vi "Path - ResolveHostRoot.vi"(8 "error in (no error)":errorcluster) -> (0 "error out":errorcluster)   [LabVIEW 2026, in "Tests.lvlib"]
doc: "Update with test documentation"
uses:
  Tests.lvlib
  <vilib>/addons/_JKI Toolkits/Caraya/classes/Assert/Assert Equal Value_Variant.vi
  <vilib>/addons/_JKI Toolkits/Caraya/classes/Assert/Assert Error.vi
  <vilib>/addons/_JKI Toolkits/Caraya/classes/Test/Test.lvclass
  src/Lumberjack.lvlib
  <vilib>/addons/_JKI Toolkits/Caraya/classes/Assert/Assert.lvclass
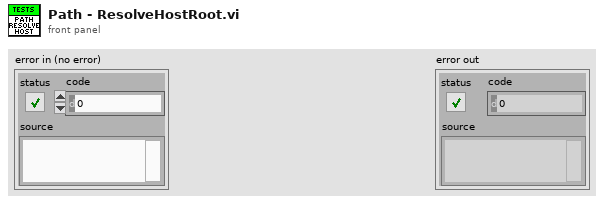
[diagram p1: front panel]
types:
  T1 = enum32{"Auto", "Development System", "Run Time System"}
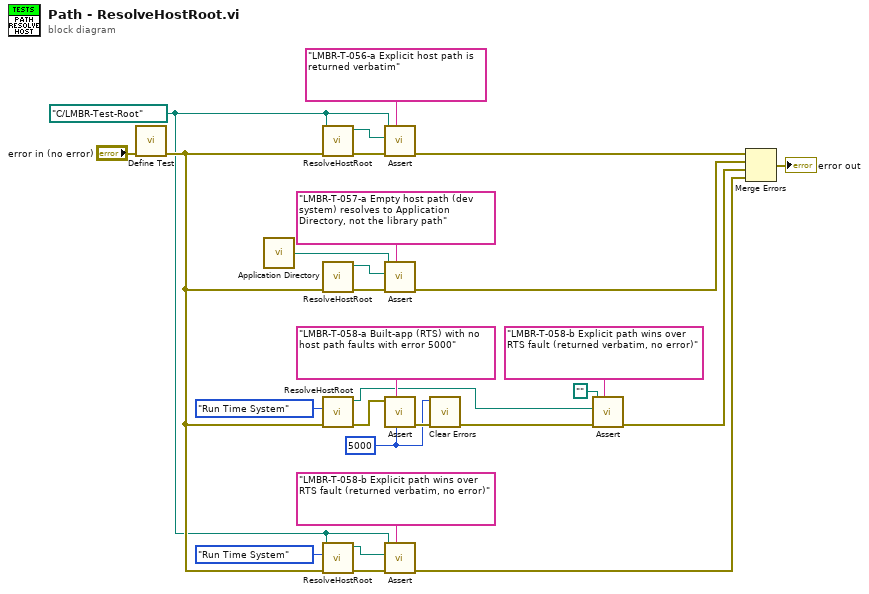
[diagram p0: block diagram]
diagram:
  w14 = 5000 ("error code (1)")
  w9 = path "C:/LMBR-Test-Root" ("HostApplicationPath")
  n1 = call <vilib>:"Define Test.vi"("error in (no error)"="error in (no error)") -> ("error out"=w11:errorcluster)  [unwired: 9 in, 1 out]
  n2 = call <vilib>:"Application Directory.vi"() -> ("Application Directory"=w19:path)
  n3 = call "ResolveHostRoot.vi"("error in (no error)"=w11, "HostApplicationPath"=w9) -> ("error out"=w25:errorcluster, "HostRoot"=w26:path)  [unwired: 8 in]
  n4 = call "ResolveHostRoot.vi"("error in (no error)"=w11) -> ("error out"=w21:errorcluster, "HostRoot"=w22:path)  [unwired: 9 in]
  n5 = call "ResolveHostRoot.vi"("error in (no error)"=w11, "Application:Kind"=T1."Run Time System") -> ("error out"=w16:errorcluster, "HostRoot"=w5:path)  [unwired: 8 in]
  n6 = call "ResolveHostRoot.vi"("error in (no error)"=w11, "Application:Kind"=T1."Run Time System", "HostApplicationPath"=w9) -> ("error out"=w10:errorcluster, "HostRoot"=w8:path)  [unwired: 7 in]
  n7 = call-poly <vilib>:"Assert.vi"("Label"="LMBR-T-056-a Explicit host path is returned verbatim", "error in (no error)"=w25, "Actual"=w26, "Expected"=w9) -> ("error out"=w24:errorcluster)  [unwired: 6 in, 1 out]
  n8 = call-poly <vilib>:"Assert.vi"("Label"="LMBR-T-057-a Empty host path (dev system) resolves to Application Directory, not the library path", "error in (no error)"=w21, "Actual"=w22, "Expected"=w19) -> ("error out"=w3:errorcluster)  [unwired: 6 in, 1 out]
  n9 = call-poly <vilib>:"Assert.vi"("error code (1)"=w14, "Label"="LMBR-T-058-a Built-app (RTS) with no host path faults with error 5000", "Error?"=w16) -> ("error out"=w15:errorcluster)  [unwired: 7 in, 1 out]
  n10 = call-poly <vilib>:"Assert.vi"("Label"="LMBR-T-058-b Explicit path wins over RTS fault (returned verbatim, no error)", "error in (no error)"=w10, "Actual"=w8, "Expected"=w9) -> ("error out"=w1:errorcluster)  [unwired: 6 in, 1 out]
  n11 = call <vilib>:"Clear Errors.vi"("error in (no error)"=w15, "specific error code to clear (0: all)"=w14) -> ("error out"=w7:errorcluster)  [unwired: 4 in, 1 out]
  n12 = call-poly <vilib>:"Assert.vi"("Label"="LMBR-T-058-b Explicit path wins over RTS fault (returned verbatim, no error)", "error in (no error)"=w7, "Actual"=w5, "Expected"=path "") -> ("error out"=w2:errorcluster)  [unwired: 6 in, 1 out]
  n13 = Merge Errors(w24, w3, w2, w1) -> (→"error out":errorcluster)
